vi "test Add with Unique Name.vi"(8 "error in":errorcluster, 11 "TestCase in":refnum<class "Scripting.lvclass">) -> (0 "error out":errorcluster, 3 "TestCase out":refnum<class "Scripting.lvclass">)   [LabVIEW 2020, in "Scripting.lvclass"]
uses:
  Scripting.lvclass
  Scripting.lvclass/Scripting.ctl
  <vilib>/addons/_JKI Toolkits/VI Tester/TestCase.llb/TestCase.lvclass
  Scripting/Ballard/Ballard ARINC 429 Scripting.lvlib
  <vilib>/NI VeriStand/Custom Device API/Custom Device API.lvlib
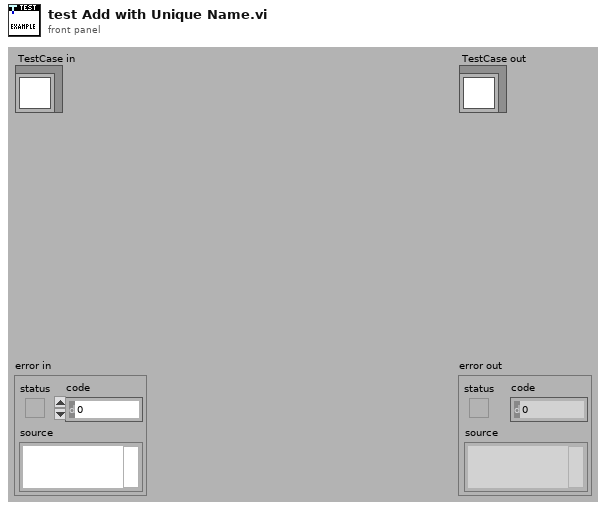
[diagram p1: front panel]
types:
  T1 = typedef "Custom Device API.lvlib/Custom Device Item Info.ctl" = cluster{"Name":string, "Is Channel":bool, "GUID":string, "Is Waveform":bool}
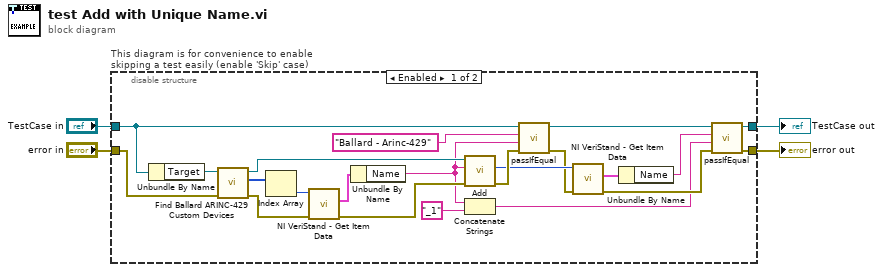
[diagram p0: block diagram]
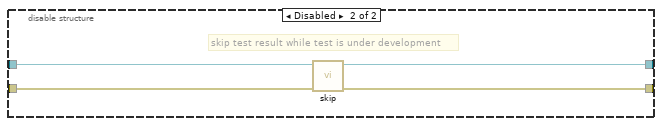
[diagram p2: hidden frame]
diagram:
  n1 = disable-structure "This diagram is for convenience to enable skipping a test easily (enable 'Skip' case)" shown="Enabled" {
    disable-tunnel: "TestCase in" -> [w25 w30]
    disable-tunnel: [w24 w28] -> w1
    disable-tunnel: [w21 w29] -> w3
    disable-tunnel: "error in" -> [w22 w27]
    frame Enabled {
      n2 = Unbundle By Name(w25) -> ("Target"=w26:refnum<k24>)
      n3 = call "Find Ballard ARINC-429 Custom Devices.vi"("error in"=w22, "target in"=w26) -> ("error out"=w18:errorcluster, "Ballard ARINC 429 custom devices"=w20:u64[], "target out"=w16:refnum<k24>)  [unwired: 7 in]
      n4 = Index Array(array=w20) -> (element=w19:u64)  [unwired: 1 in]
      n5 = call <vilib>:"NI VeriStand - Get Item Data.vi"("error in (no error)"=w18, "Item Ref in"=w19) -> ("error out"=w15:errorcluster, "Item Info"=w17:T1)  [unwired: 6 in, 2 out]
      n6 = Unbundle By Name(w17) -> ("Name"=w5:string)
      n7 = call "Add.vi"("error in"=w15, "name"=w5, "target in"=w16) -> ("error out"=w14:errorcluster, "Ballard ARINC 429 custom device"=w13:u64)  [unwired: 6 in, 1 out]
      n8 = Concatenate Strings(w5, "_1" ("string")) -> (w7:string)
      n9 = call-dynamic "passIfEqual.vi"("error in (no error)"=w14, "y"=w5, "x"="Ballard - Arinc-429" ("string"), "TestCase in"=w25) -> ("error out"=w12:errorcluster, "TestCase out"=w23:refnum<class "Scripting.lvclass">)  [unwired: 6 in]
      n10 = call <vilib>:"NI VeriStand - Get Item Data.vi"("error in (no error)"=w12, "Item Ref in"=w13) -> ("error out"=w10:errorcluster, "Item Info"=w11:T1)  [unwired: 6 in, 2 out]
      n11 = Unbundle By Name(w11) -> ("Name"=w9:string)
      n12 = call-dynamic "passIfEqual.vi"("error in (no error)"=w10, "y"=w7, "x"=w9, "TestCase in"=w23) -> ("error out"=w21:errorcluster, "TestCase out"=w24:refnum<class "Scripting.lvclass">)  [unwired: 6 in]
    }
    frame Disabled {
      # "skip test result while test is under development"
      n13 = call <vilib>:"skip.vi"("error in (no error)"=w27, "TestCase in"=w30) -> ("error out"=w29:errorcluster, "TestCase out"=w28:refnum<class "Scripting.lvclass">)  [unwired: 8 in]
    }
  }
  "error out" <- w3
  "TestCase out" <- w1
